vi "XY Graph Compute Plots Circular Convolution Product v3.vi"(8 "Error In":errorcluster, 9 "Support Axis (kernel's)":dbl[](array[numeric]), 10 "Plot 2 (kernel)":T1, 11 "Plot 1 (function)":T1) -> (0 "Error Out":errorcluster, 1 "CPU (s)":dbl, 3 "Convolution Product":T1)   [LabVIEW 2021, in "XY Graph Add-Ons.lvlib"]
doc: "Convolves two plots interpolated over the provided <B>Support Axis</b>.\n\nIf <B>Support Axis</B> is empty, uses the support of <B>Plot 2</B> considered as the <B>kernel</B> for the convolution product (otherwise both plots have an identical role)."
uses:
  XY Graph Add-Ons.lvlib
  XY Plot Data.ctl
  Time/Time.lvlib
  Math/Math.lvlib
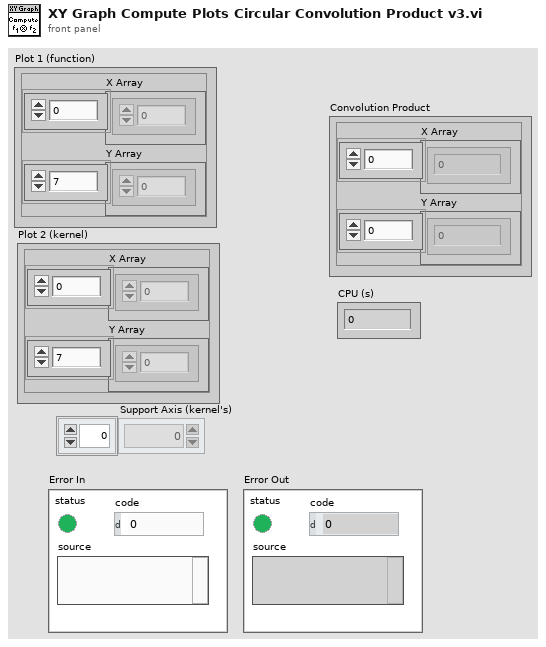
[diagram p1: front panel]
types:
  T1 = typedef "XY Graph Add-Ons.lvlib/XY Plot Data.ctl" = cluster{"X Array":dbl[], "Y Array":dbl[]}
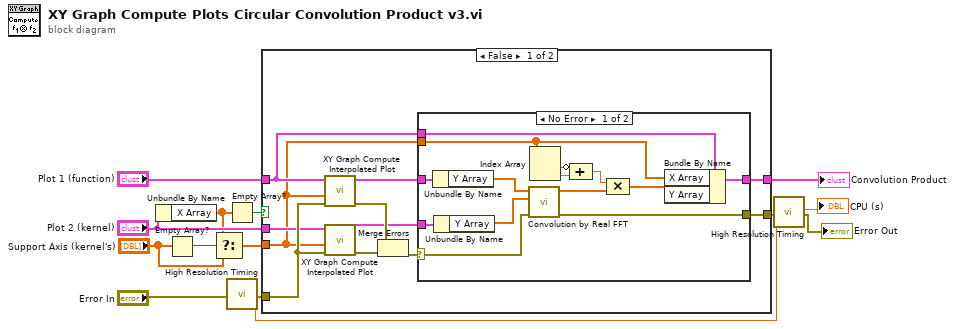
[diagram p0: block diagram]
diagram:
  n1 = Unbundle By Name("Plot 2 (kernel)") -> ("X Array"=w3:dbl[])
  n2 = Empty Array?(array="Support Axis (kernel's)") -> (empty?=w6:bool)
  n3 = Select(t=w3, s=w6, f="Support Axis (kernel's)") -> (s? t:f=w4:dbl[])
  n4 = Empty Array?(array=w3) -> (empty?=w2:bool)
  n5 = call "High Resolution Timing.vi"("Error In"="Error In") -> ("elapsed (relative) seconds"=w1:dbl, "Error Out"=w8:errorcluster)  [unwired: 16 in, 1 out]
  n6 = case shown="False" w2 {
    tunnel: [w25 w43] -> w13
    tunnel: "Plot 1 (function)" -> [w24 w43]
    tunnel: [w20 w42] -> w11
    tunnel: w8 -> [w17 w42]
    tunnel: "Plot 2 (kernel)" -> [w16 _]
    tunnel: w4 -> [w15 _]
    frame False {
      n7 = call "XY Graph Compute Interpolated Plot.vi"("Error In"=w17, "Ramp"=w15, "Plot"=w24) -> ("Error Out"=w22:errorcluster, "Interpolated Plot"=w23:T1)  [unwired: 7 in]
      n8 = call "XY Graph Compute Interpolated Plot.vi"("Error In"=w17, "Ramp"=w15, "Plot"=w16) -> ("Error Out"=w19:errorcluster, "Interpolated Plot"=w18:T1)  [unwired: 7 in]
      n9 = Merge Errors(w22, w19) -> (w21:errorcluster)
      n10 = case shown="No Error" w21 {
        selector: w21 -> [w31 w41]
        tunnel: [w38 w40] -> w25
        tunnel: w24 -> [w37 w40]
        tunnel: w15 -> [w29 _]
        tunnel: w23 -> [w36 _]
        tunnel: w18 -> [w34 _]
        tunnel: [w30 w41] -> w20
        frame No Error {
          n11 = Unbundle By Name(w36) -> ("Y Array"=w35:dbl[])
          n12 = Unbundle By Name(w34) -> ("Y Array"=w33:dbl[])
          n13 = call "Convolution by Real FFT.vi"("error in (no error)"=w31, "Array 2"=w33, "Array 1"=w35) -> ("error out"=w30:errorcluster, "Convolution"=w32:dbl[])  [unwired: 7 in]
          n14 = Index Array(array=w29) -> (element #1=w28:dbl, element #2=w27:dbl)  [unwired: 2 in]
          n15 = Compound Arithmetic op=ADD(invert w28, w27) -> (w26:dbl)
          n16 = Compound Arithmetic op=MULTIPLY(w26, w32) -> (w39:dbl[])
          n17 = Bundle By Name(cluster=w37, "X Array"=w29, "Y Array"=w39) -> (w38:T1)
        }
        frame Error {
        }
      }
    }
    frame True {
      # "empty kernel: skip convolution"
    }
  }
  "Convolution Product" <- w13
  n18 = call "High Resolution Timing.vi"("relative seconds (NaN)"=w1, "Error In"=w11) -> ("elapsed (relative) seconds"=→"CPU (s)":dbl, "Error Out"=→"Error Out":errorcluster)  [unwired: 15 in, 1 out]
